vi "Read_Parameters.vi"(10 "error in":errorcluster, 11 "device count":u8) -> (1 "error out":errorcluster, 2 "Selected Devices":i32, 3 "Device Configuration":T1(array[cluster]))   [LabVIEW 2026]
uses:
  Include/DEVICE_CONFIG_PARAM.ctl
panel:
  out "Number of Devices":string[](array[string])
  out "Status":string[](array[string])
  out "Baud Rate":i32
  out "CAN FD Bitrate":i32
  out "Configure Devices":string[](array[string])
  out "Baud Rate 2":string="Baud Rate Selected Successfully"
  out "Baud Rate":string="Baud Rate Selected Successfully"
  in  "DEVICE CONFIG PARAMETERS":T2
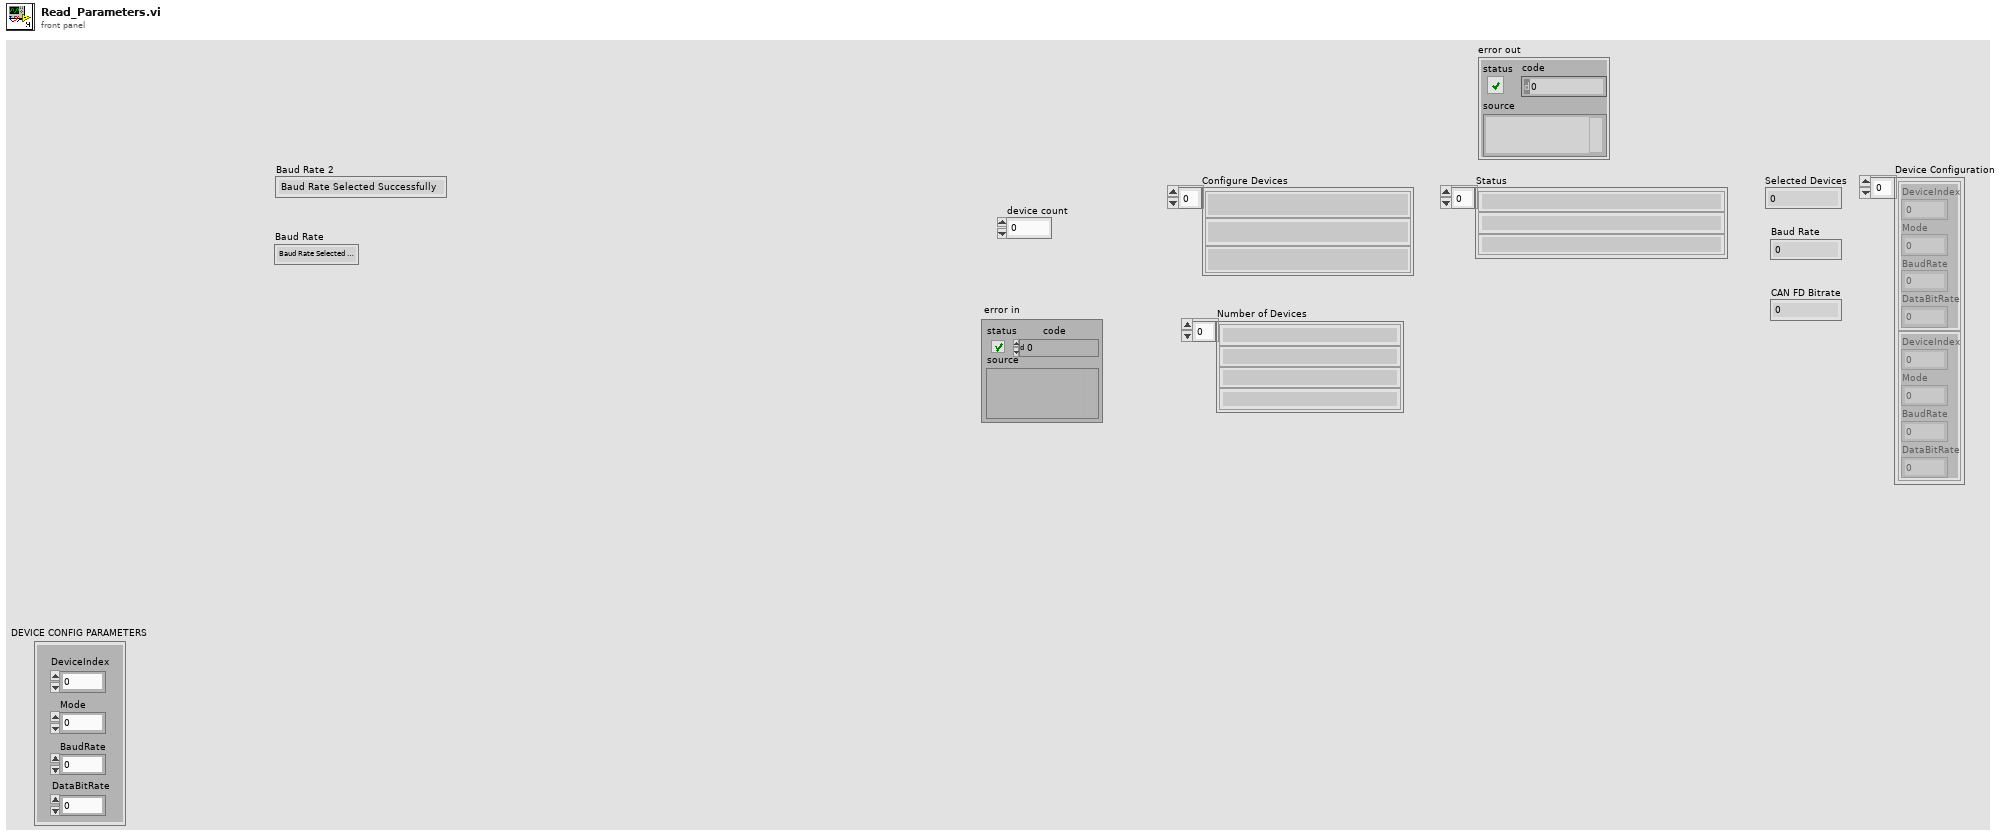
[diagram p1: front panel]
types:
  T1 = cluster{"DeviceIndex":i32, "Mode":i32, "BaudRate":i32, "DataBitRate":i32}[]
  T2 = typedef "DEVICE_CONFIG_PARAM.ctl" = cluster{"DeviceIndex":i32, "Mode":i32, "BaudRate":i32, "DataBitRate":i32}
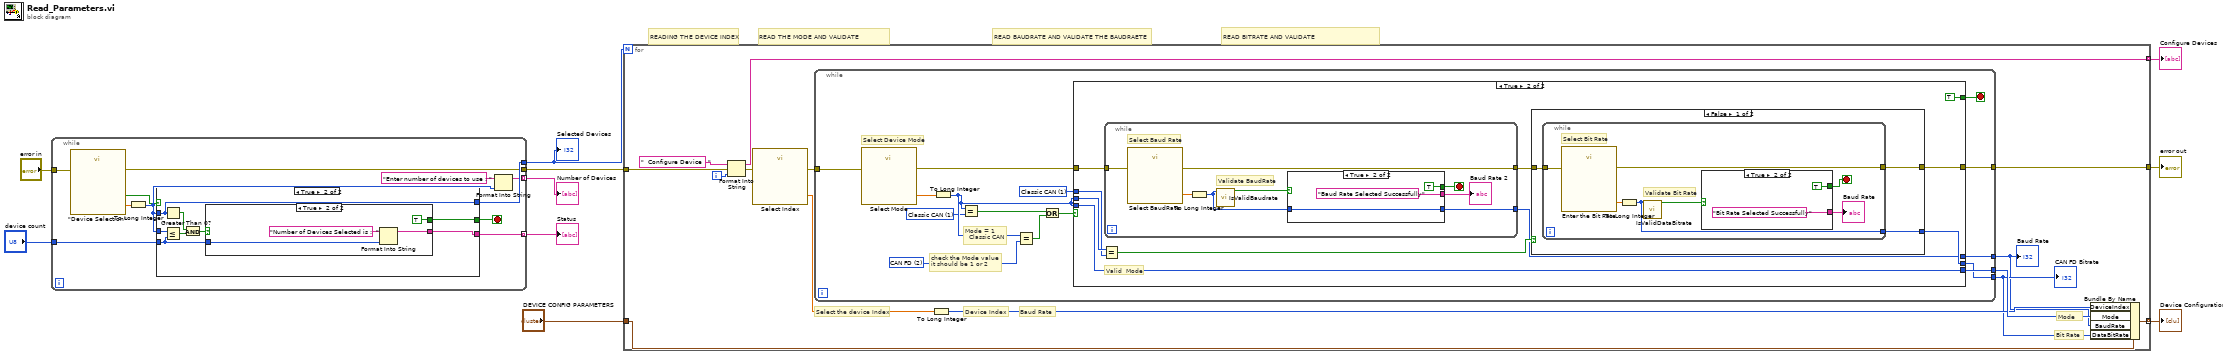
[diagram p0: block diagram]
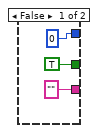
[diagram p2: hidden frame]
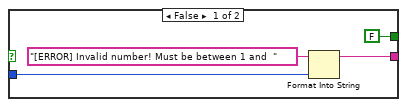
[diagram p3: hidden frame]
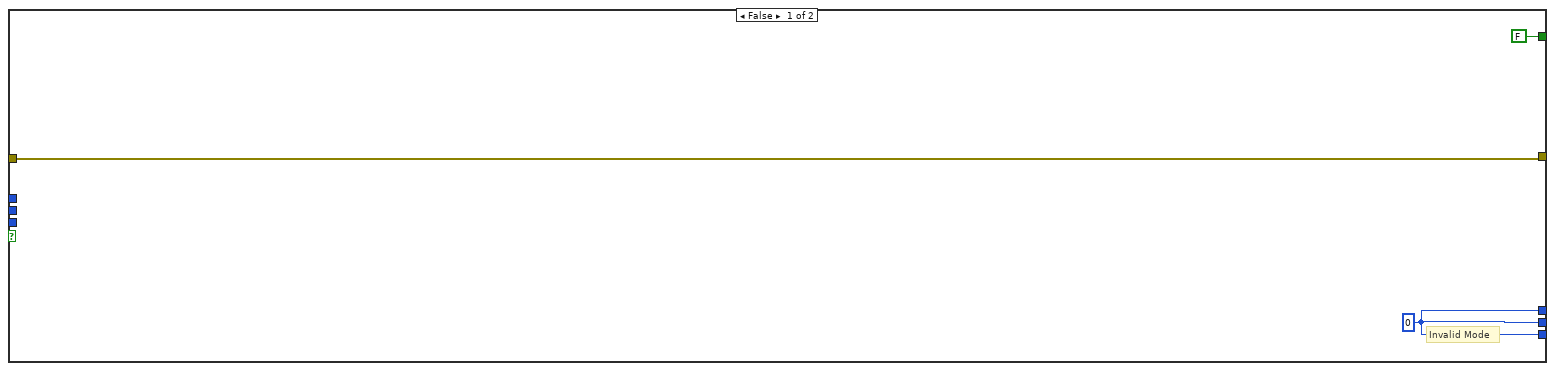
[diagram p4: hidden frame]
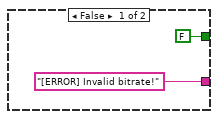
[diagram p5: hidden frame]
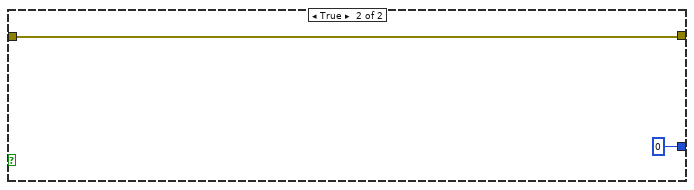
[diagram p6: hidden frame]
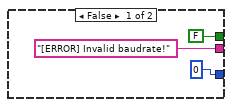
[diagram p7: hidden frame]
diagram:
  # "READ BITRATE AND VALIDATE"
  # "READ BAUDRATE AND VALIDATE THE BAUDRAETE"
  # "READ THE MODE AND VALIDATE"
  # "READING THE DEVICE INDEX"
  n1 = while {
    tunnel: "device count" -> [w20]
    tunnel: [w19] -> w7 mode=indexing
    tunnel: [w16] -> w2
    tunnel: [w14] -> w6 mode=indexing
    tunnel: [w13] -> w3
    tunnel: "error in" -> [w11]
    stop <- w18 stop-if-true
    n2 = call "\"Device Selection\""("error in (no error)"=w11) -> ("\"Device Count\""=w15:dbl, "OK"=w21:bool, "error out"=w13:errorcluster)  [unwired: 16 in]
    n3 = To Long Integer(number=w15) -> (32bit integer=w12:i32)
    n4 = case shown="True" w21 {
      tunnel: w12 -> [_ w25]
      tunnel: w12 -> [_ w30]
      tunnel: w20 -> [_ w28]
      tunnel: [TRUE w27] -> w18
      tunnel: ["" w26] -> w19
      tunnel: [0 w25] -> w16
      frame False {
      }
      frame True {
        n5 = Greater Than 0?(x=w25) -> (x > 0?=w31:bool)
        n6 = Less Or Equal?(x=w30, y=w28) -> (x <= y?=w32:bool)
        n7 = And(x=w31, y=w32) -> (x .and. y?=w29:bool)
        n8 = case shown="True" w29 {
          tunnel: w28 -> [w36 w39]
          tunnel: [FALSE TRUE] -> w27
          tunnel: [w33 w37] -> w26
          frame False {
            n9 = Format Into String(initial string="[ERROR] Invalid number! Must be between 1 and  ", w36) -> (resulting string=w33:string)  [unwired: 2 in, 1 out]
          }
          frame True {
            n10 = Format Into String(initial string="Number of Devices Selected is :  ", w39) -> (resulting string=w37:string)  [unwired: 2 in, 1 out]
          }
        }
      }
    }
    n11 = Format Into String(initial string="Enter number of devices to use : ", w12) -> (resulting string=w14:string)  [unwired: 2 in, 1 out]
  }
  "Status" <- w7
  "Number of Devices" <- w6
  "Selected Devices" <- w2
  n12 = for {
    N: w2 -> [_]
    tunnel: [w52] -> w10 mode=indexing
    tunnel: [w47] -> w9 mode=indexing
    tunnel: w3 -> [w46]
    tunnel: "DEVICE CONFIG PARAMETERS" -> [w43]
    tunnel: [w41] -> w1
    i -> [w53]
    # "Select the device Index"
    # "Bit Rate"
    # "Mode"
    # "Baud Rate"
    # "Device Index"
    n13 = Format Into String(initial string="  Configure Device   ", error in=w46, w53) -> (resulting string=w52:string, error out=w51:errorcluster)  [unwired: 1 in]
    n14 = call "Select Index"("error in (no error)"=w51) -> ("index"=w50:dbl, "error out"=w42:errorcluster)  [unwired: 16 in, 1 out]
    n15 = while {
      tunnel: w42 -> [w68]
      tunnel: [w62] -> w49
      tunnel: [w60] -> w44
      tunnel: [w59] -> w45
      tunnel: [w55] -> w41
      stop <- w67 stop-if-true
      w56 = u16 2 items=["Classic CAN"=1, "CAN FD"=2] ("Mode")
      w57 = u16 1 items=["Classic CAN"=1, "CAN FD"=2] ("Mode")
      w58 = u16 1 items=["Classic CAN"=1, "CAN FD"=2] ("Mode")
      # "Mode = 1\n  Classic CAN"
      # "check the Mode value\nit should be 1 or 2"
      # "Select Device Mode"
      n16 = call "Select Mode"("error in (no error)"=w68) -> ("Mode"=w69:dbl, "error out"=w63:errorcluster)  [unwired: 16 in, 1 out]
      n17 = To Long Integer(number=w69) -> (32bit integer=w61:i32)
      n18 = Equal?(x=w61, y=w57) -> (x = y?=w66:bool)
      n19 = Equal?(x=w61, y=w56) -> (x = y?=w65:bool)
      n20 = Or(x=w66, y=w65) -> (x .or. y?=w64:bool)
      n21 = case shown="True" w64 {
        tunnel: [FALSE TRUE] -> w67
        tunnel: w63 -> [w70 w81]
        tunnel: w61 -> [_ w80]
        tunnel: [w71 w77] -> w62
        tunnel: w61 -> [_ w77]
        tunnel: [w71 w74] -> w60
        tunnel: [w71 w76] -> w59
        tunnel: w58 -> [_ w75]
        tunnel: [w70 w73] -> w55
        frame False {
          w71 = 0
          # "Invalid Mode"
        }
        frame True {
          # "Valid  Mode"
          n22 = Equal?(x=w80, y=w75) -> (x = y?=w79:bool)
          n23 = while {
            tunnel: w81 -> [w106]
            tunnel: [w103] -> w78
            tunnel: [w101] -> w74
            stop <- w104 stop-if-true
            # "Validate BaudRate"
            # "Select Baud Rate"
            n24 = call "Select BaudRate"("error in (no error)"=w106) -> ("BaudRate"=w102:dbl, "error out"=w103:errorcluster)  [unwired: 16 in, 1 out]
            n25 = To Long Integer(number=w102) -> (32bit integer=w100:i32)
            n26 = call "IsValidBaudrate.vi"("Baud Rate"=w100) -> ("x >= 0?"=w99:bool)  [unwired: 10 in]
            n27 = case shown="True" w99 {
              tunnel: ["[ERROR] Invalid baudrate!" "Baud Rate Selected Successfully"] -> w105
              tunnel: [FALSE TRUE] -> w104
              tunnel: [0 w110] -> w101
              tunnel: w100 -> [_ w110]
              frame False {
              }
              frame True {
              }
            }
            "Baud Rate 2" <- w105
          }
          n28 = case shown="False" w79 {
            tunnel: w78 -> [w85 w97]
            tunnel: [w84 0] -> w76
            tunnel: [w83 w97] -> w73
            frame False {
              n29 = while {
                tunnel: w85 -> [w89]
                tunnel: [w88] -> w84
                tunnel: [w86] -> w83
                stop <- w90 stop-if-true
                # "Validate Bit Rate"
                # "Select Bit Rate"
                n30 = call "Enter the Bit Rate"("error in (no error)"=w89) -> ("BitRate"=w92:dbl, "error out"=w86:errorcluster)  [unwired: 16 in, 1 out]
                n31 = To Long Integer(number=w92) -> (32bit integer=w88:i32)
                n32 = call "IsValidDataBitrate.vi"("Bit Rate"=w88) -> ("x >= 0?"=w87:bool)  [unwired: 10 in]
                n33 = case shown="True" w87 {
                  tunnel: ["[ERROR] Invalid bitrate!" "Bit Rate Selected Successfully"] -> w91
                  tunnel: [FALSE TRUE] -> w90
                  frame False {
                  }
                  frame True {
                  }
                }
                "Baud Rate" <- w91
              }
            }
            frame True {
            }
          }
        }
      }
    }
    "CAN FD Bitrate" <- w45
    "Baud Rate" <- w44
    n34 = To Long Integer(number=w50) -> (32bit integer=w48:i32)
    n35 = Bundle By Name(cluster=w43, "DeviceIndex"=w48, "Mode"=w49, "BaudRate"=w44, "DataBitRate"=w45) -> (w47:T2)
  }
  "Configure Devices" <- w10
  "Device Configuration" <- w9
  "error out" <- w1
